vi "ballPathWithAir.vi"() -> ()   [LabVIEW 2017]
panel:
  out "轨迹":cluster{dbl[], dbl[]}(graph)
  in  "停止":bool
  in  "时间细分":dbl=0.01
  in  "时间长度":dbl(slide) scale=0.0..5.0
  in  "角度":dbl(slide) scale=0.0..90.0
  in  "速度":dbl(slide) scale=0.0..20.0
  # "篮球轨迹计算"
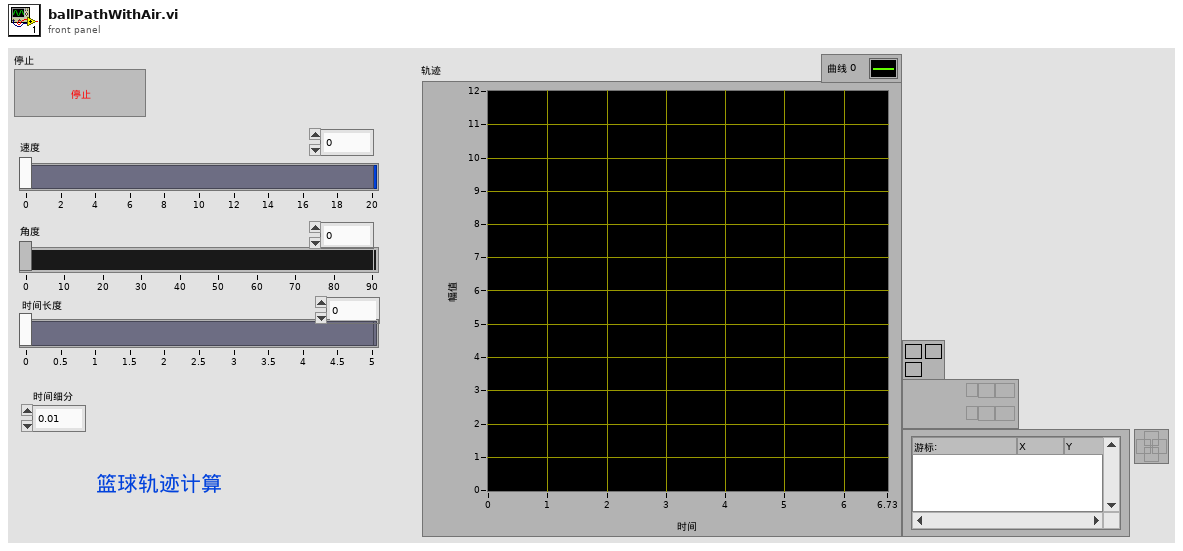
[diagram p1: front panel]
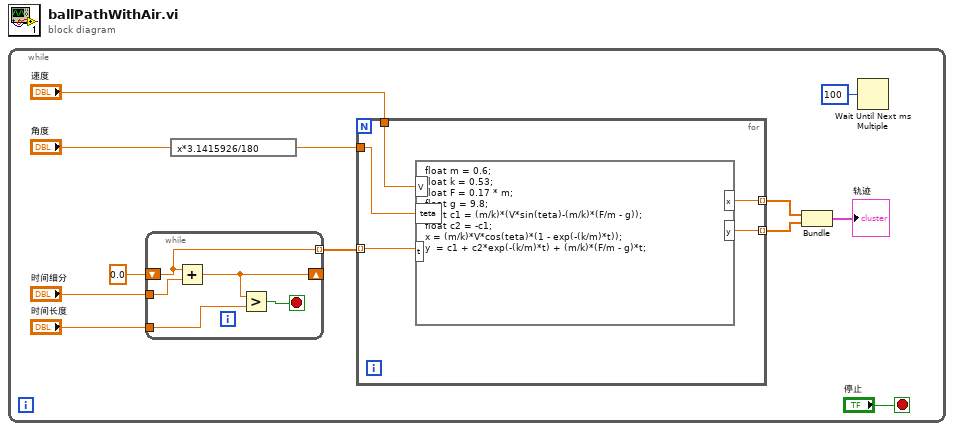
[diagram p0: block diagram]
diagram:
  n1 = while {
    stop <- "停止" stop-if-true
    n2 = while {
      shift-right: [w20] -> _
      shift-left: 0.0 -> [w21]
      tunnel: "时间细分" -> [w22]
      tunnel: [w21] -> w8 mode=indexing
      tunnel: "时间长度" -> [w19]
      stop <- w18 stop-if-true
      n3 = Add(x=w21, y=w22) -> (x+y=w20:dbl)
      n4 = Greater?(x=w20, y=w19) -> (0:w18:bool)
    }
    n5 = expression code="x*3.1415926/180"("角度") -> (w5:dbl)
    n6 = for {
      tunnel: "速度" -> [w17]
      tunnel: w5 -> [w16]
      tunnel: w8 -> [w15] mode=indexing
      tunnel: [w14] -> w7 mode=indexing
      tunnel: [w13] -> w6 mode=indexing
      n7 = formula code="float m = 0.6;\nfloat k = 0.53;\nfloat F = 0.17 * m;\nfloat g = 9.8;\nfloat c1 = (m/k)*(V*sin(teta)-(m/k)*(F/m - g));\nfloat c2 = -c1;\nx = (m/k)*V*cos(teta)*(1 - exp(-(k/m)*t));\ny  = c1 + c2*exp(-(k/m)*t) + (m/k)*(F/m - g)*t;"("V"=w17, "teta"=w16, "t"=w15) -> ("x"=w14:dbl, "y"=w13:dbl)
    }
    n8 = Bundle(w7, w6) -> (→"轨迹":cluster{dbl[], dbl[]})  [unwired: 1 in]
    n9 = Wait Until Next ms Multiple(millisecond multiple=u32 100 ("毫秒倍数")) -> ()  [unwired: 1 out]
  }
